vi "error_report.vi"(8 "_Frame Rate":dbl, 9 "frame #":i32, 10 "# of frame":i32, 11 "refnum":refnum<file>) -> (0 "error out":errorcluster, 2 "refnum out":refnum<file>)   [LabVIEW 2015]
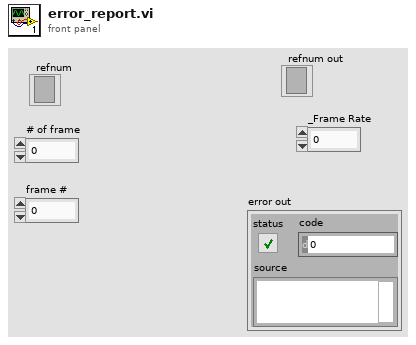
[diagram p1: front panel]
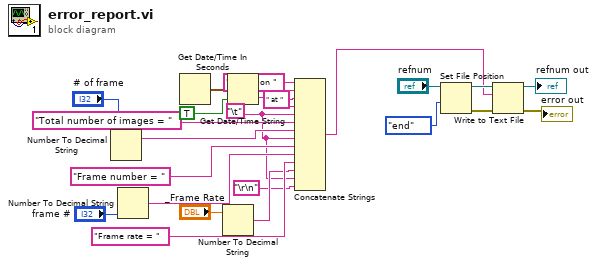
[diagram p0: block diagram]
diagram:
  w1 = "\t"
  n1 = Number To Decimal String(number="# of frame") -> (decimal integer string=w13:string)  [unwired: 1 in]
  n2 = Number To Decimal String(number="frame #") -> (decimal integer string=w4:string)  [unwired: 1 in]
  n3 = Get Date/Time In Seconds() -> (seconds since 1Jan1904=w24:timestamp)
  n4 = Number To Decimal String(number="_Frame Rate") -> (decimal integer string=w5:string)  [unwired: 1 in]
  n5 = Get Date/Time String(seconds (now)=w24, want seconds? (F)=TRUE) -> (date string=w18:string, time string=w16:string)  [unwired: 1 in]
  n6 = Concatenate Strings("Freeze on " ("string"), w18, " at " ("string"), w16, w1, "Total number of images = " ("string"), w13, w1, "Frame number = " ("string"), w4, "Frame rate = " ("string"), w5, w1, "\r\n") -> (w19:string)
  n7 = Set File Position(refnum="refnum", from (0:start)=enum16{"start", "end", "current"}."end") -> (refnum out=w20:refnum<file>, error out=w21:errorcluster)  [unwired: 2 in]
  n8 = Write to Text File(file (use dialog)=w20, text=w19, error in=w21) -> (refnum out=→"refnum out":refnum<file>, error out=→"error out":errorcluster)  [unwired: 1 in, 1 out]
